vi "process_checkin.vi"(8 "error in (no error)":errorcluster, 9 "library map in":T1, 10 "message":T5, 11 "client map in":T4(c390)) -> (0 "error out":errorcluster, 1 "state":string, 2 "library map out":T1, 3 "client map out":T4(c390))   [LabVIEW 2020, in "librarian.lvclass"]
uses:
  librarian.lvclass
  typedefs/library--map.ctl
  typedefs/lib_map_value--cluster.ctl
  typedefs/book_state--enum.ctl
  shared/message--cluster.ctl
  shared/request--enum.ctl
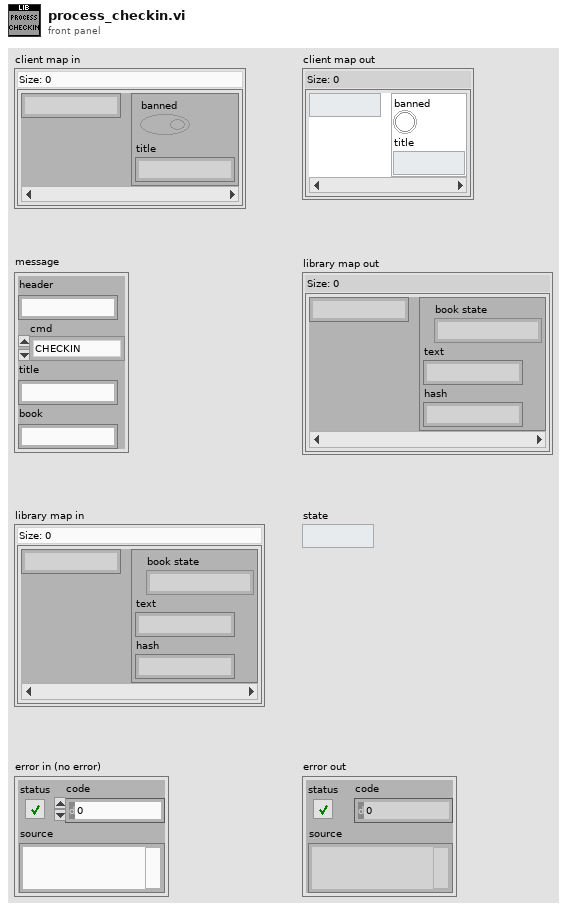
[diagram p1: front panel]
types:
  T1 = typedef "librarian.lvclass/library--map.ctl" = map{string, T2}
  T2 = typedef "librarian.lvclass/lib_map_value--cluster.ctl" = cluster{"book state":T3, "text":string, "hash":string}
  T3 = typedef "librarian.lvclass/book_state--enum.ctl" = enum16{"CHECKEDIN", "CHECKEDOUT", "DAMAGED"}
  T4 = map{string, cluster{"banned":bool, "title":string}}
  T5 = typedef "message--cluster.ctl" = cluster{"header":string, "cmd":T6, "title":string, "book":string}
  T6 = typedef "request--enum.ctl" = enum16{"CHECKIN", "CHECKOUT"}
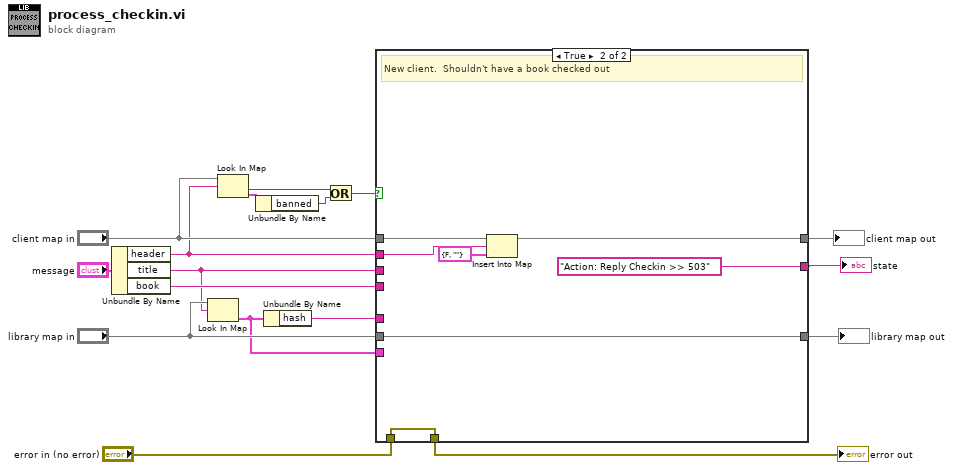
[diagram p0: block diagram]
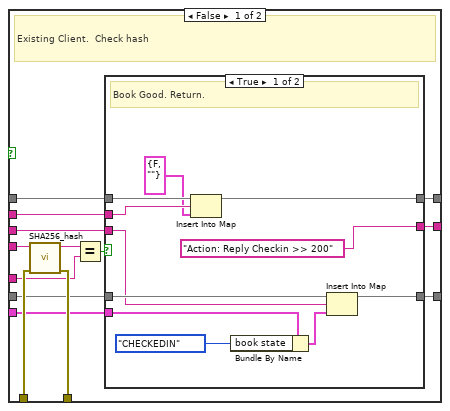
[diagram p2: hidden frame]
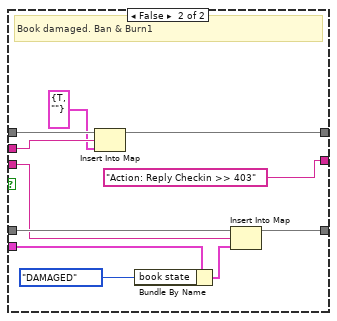
[diagram p3: hidden frame]
diagram:
  n1 = Unbundle By Name("message") -> ("header"=w2:string, "title"=w1:string, "book"=w11:string)
  n2 = Look In Map(map="library map in", key=w1) -> (value=w8:T2)  [unwired: 1 in, 1 out]
  n3 = Look In Map(map="client map in", key=w2) -> (key not found?=w15:bool, value=w17:cluster{"banned":bool, "title":string})  [unwired: 1 in]
  n4 = Unbundle By Name(w17) -> ("banned"=w16:bool)
  n5 = Unbundle By Name(w8) -> ("hash"=w9:string)
  n6 = Or(x=w15, y=w16) -> (x .or. y?=w12:bool)
  n7 = case shown="True" w12 {
    tunnel: w1 -> [w20 _]
    tunnel: w2 -> [w24 w58]
    tunnel: "client map in" -> [w25 w59]
    tunnel: [w18 "Action: Reply Checkin >> 503"] -> w4
    tunnel: [w23 w56] -> w5
    tunnel: w9 -> [w27 _]
    tunnel: w11 -> [w31 _]
    tunnel: "error in (no error)" -> [w30 w55]
    tunnel: [w29 w55] -> w6
    tunnel: "library map in" -> [w22 w54]
    tunnel: [w21 w54] -> w3
    tunnel: w8 -> [w19 _]
    frame False {
      # "Existing Client.  Check hash"
      n8 = call "SHA256_hash.vi"("error in (no error)"=w30, "text in"=w31) -> ("error out"=w29:errorcluster, "hash out"=w28:string)  [unwired: 8 in]
      n9 = Equal?(x=w28, y=w27) -> (x = y?=w26:bool)
      n10 = case shown="True" w26 {
        tunnel: w25 -> [w42 w53]
        tunnel: w24 -> [w40 w51]
        tunnel: [w41 w52] -> w23
        tunnel: w22 -> [w38 w49]
        tunnel: [w37 w48] -> w21
        tunnel: w20 -> [w33 w44]
        tunnel: w19 -> [w36 w47]
        tunnel: ["Action: Reply Checkin >> 200" "Action: Reply Checkin >> 403"] -> w18
        frame True {
          # "Book Good. Return."
          n11 = Insert Into Map(map in=w42, key=w40, value=cluster{"banned":bool, "title":string} {"banned"=FALSE, "title"=""}) -> (map out=w41:T4)  [unwired: 2 out]
          n12 = Bundle By Name(cluster=w36, "book state"=book_state--enum."CHECKEDIN") -> (w34:T2)
          n13 = Insert Into Map(map in=w38, key=w33, value=w34) -> (map out=w37:T1)  [unwired: 2 out]
        }
        frame False {
          # "Book damaged. Ban & Burn1"
          n14 = Insert Into Map(map in=w53, key=w51, value=cluster{"banned":bool, "title":string} {"banned"=TRUE, "title"=""}) -> (map out=w52:T4)  [unwired: 2 out]
          n15 = Bundle By Name(cluster=w47, "book state"=book_state--enum."DAMAGED") -> (w45:T2)
          n16 = Insert Into Map(map in=w49, key=w44, value=w45) -> (map out=w48:T1)  [unwired: 2 out]
        }
      }
    }
    frame True {
      # "New client.  Shouldn't have a book checked out"
      n17 = Insert Into Map(map in=w59, key=w58, value=cluster{"banned":bool, "title":string} {"banned"=FALSE, "title"=""}) -> (map out=w56:T4)  [unwired: 2 out]
    }
  }
  "error out" <- w6
  "client map out" <- w5
  "state" <- w4
  "library map out" <- w3
